vi "Process Incoming Messages by PDU F.vi"(0 "J1939 Cluster":T11, 1 "Conv Ref":T2, 2 "Data Ref":T1, 5 "CAN frame":T9 {"payload" format="%x"; "timestamp" format="%<%.7X\n%x>T"; "type" items=["CAN Data"=0, "CAN Remote"=1, "CAN Bus Error"=2, "Delay"=224, "Log Trigger"=225, "Start Trigger"=226]; "identifier" format="%x"}, 7 "ref in":T3, 9 "Addresses":u8[](array[numeric]), 11 "error in":errorcluster, 12 "Simulated Addresses LUT":variant) -> (15 "error out":errorcluster)   [LabVIEW 2013, in "J1939 Addon Engine.lvlib"]
uses:
  Engine/J1939 Addon Engine.lvlib
  Types/Setup Information Cluster.ctl
  <vilib>/xnet/xnet.llb/XNET Frame CAN.ctl
  <vilib>/xnet/xnet.llb/XNET Frame Type CAN.ctl
  J1939 Utilities/Types/CAN Outgoing Message Cluster.ctl
  Types/TP List References.ctl
  Types/BAM Buffer Connections List_Ref.ctl
  Types/Connection Mode Generation Connection Ref.ctl
  Types/BAM Generation Connections List_Ref.ctl
  Types/Address Table Reference.ctl
  Types/RQST Lookup Table Reference.ctl
  Engine/Types/Conversion Lookup Table Reference.ctl
  Engine/Types/Data Lookup Table Reference.ctl
  J1939 Utilities/Types/PGN Fields Cluster.ctl
  Engine/Types/Simulated Settings.ctl
  Types/Compiled Simulated Settings.ctl
  Types/Monitor Settings.ctl
  <vilib>/NI Veristand/Custom Device API/Block Data Reference.ctl
  <vilib>/NI Veristand/Custom Device API/Data Reference.ctl
  Engine/Types/DTC FIFOs.ctl
  Types/TP Connections List State.ctl
  Types/Connection Mode Buffer Create New TP Connection State.ctl
  Types/Address Lookup Table Action.ctl
  Types/Address Lookup Table Data.ctl
  J1939 Utilities/SubVIs/Convert CAN Arb ID to J1939 ID.vi
  J1939 Utilities/SubVIs/Convert J1939 ID to CAN Arb ID.vi
  J1939 Utilities/SubVIs/Acknowledgement.vi
  Buffer Connections List_Actions.vi
  TP Buffer Search for Connection (No PGN).vi
  TP Buffer Add New Data Packet to Connection.vi
  TP Buffer Convert Connection Info to CAN Frame.vi
  TP Buffer Create New TP Connection.vi
  Connection Mode Generation Connections List_Actions.vi
  Connection Mode Generation Search for Connection (Remote Message).vi
  TP Buffer Search for Connection.vi
  Engine/SubVIs/Convert Data to DTC Frame.vi
  Engine/SubVIs/Conversion Lookup Table Get Conversion Parameter.vi
  Engine/SubVIs/Data Lookup Table Get Signals (Range).vi
  J1939 Utilities/SubVIs/Convert PGN + SA to J1939 ID.vi
  <vilib>/xnet/xnet.llb/XNET Convert.vi
  <vilib>/xnet/xnet.llb/XNET Convert (Signal to Frame Raw).vi
  J1939 Utilities/SubVIs/TP.CM EndofMsgACK.vi
  J1939 Utilities/SubVIs/TP.CM CTS.vi
  J1939 Utilities/SubVIs/TP.Conn Abort.vi
  Connection Mode Generation CTS Received.vi
  J1939 Utilities/SubVIs/Convert CAN Data (U32) to U8.vi
  J1939 Utilities/J1939 Utilities.lvlib
  J1939 Addon Shared.lvlib
  <vilib>/NI Veristand/Custom Device API/Custom Device API.lvlib
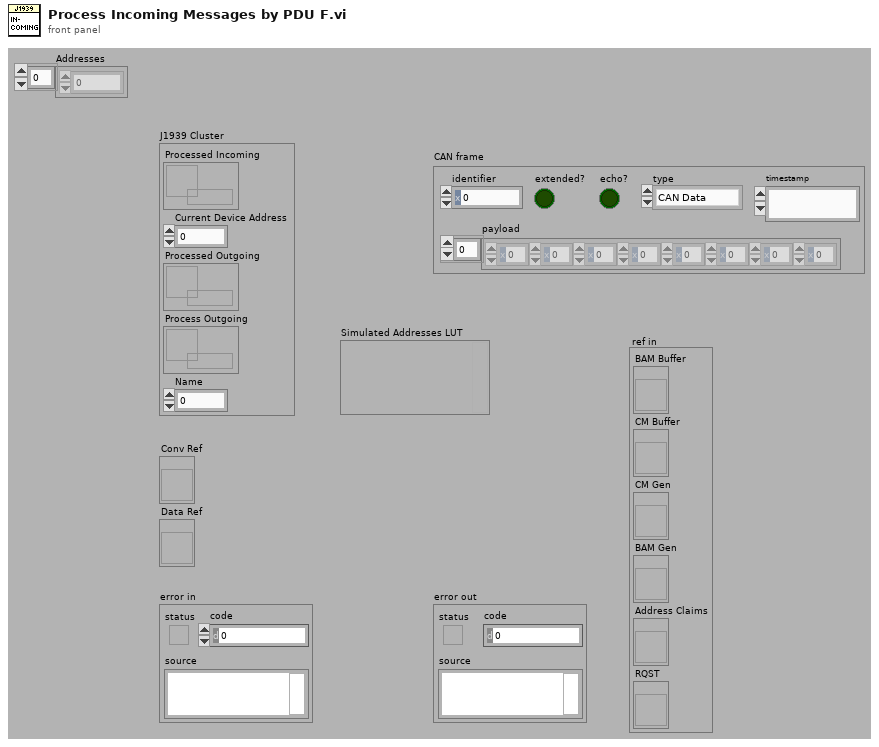
[diagram p1: front panel]
types:
  T1 = typedef "J1939 Addon Engine.lvlib/Data Lookup Table Reference.ctl" = refnum<vi>
  T2 = typedef "J1939 Addon Engine.lvlib/Conversion Lookup Table Reference.ctl" = refnum<vi>
  T3 = typedef "J1939 Addon Engine.lvlib/TP List References.ctl" = cluster{"BAM Buffer":T4, "CM Buffer":T4, "CM Gen":T5, "BAM Gen":T6, "Address Claims":T7, "RQST":T8}
  T4 = typedef "J1939 Addon Engine.lvlib/BAM Buffer Connections List_Ref.ctl" = refnum<vi>
  T5 = typedef "J1939 Addon Engine.lvlib/Connection Mode Generation Connection Ref.ctl" = refnum<vi>
  T6 = typedef "J1939 Addon Engine.lvlib/BAM Generation Connections List_Ref.ctl" = refnum<vi>
  T7 = typedef "J1939 Addon Engine.lvlib/Address Table Reference.ctl" = refnum<vi>
  T8 = typedef "J1939 Addon Engine.lvlib/RQST Lookup Table Reference.ctl" = refnum<vi>
  T9 = typedef "XNET Frame CAN.ctl" = cluster{"timestamp":timestamp, "payload":u8[], "identifier":u32, "type":T10, "extended?":bool, "echo?":bool}
  T10 = typedef "XNET Frame Type CAN.ctl" = u8
  T11 = typedef "J1939 Addon Engine.lvlib/Setup Information Cluster.ctl" = cluster{"Processed Incoming":refnum<queue>, "Current Device Address":u8, "Processed Outgoing":refnum<queue>, "Process Outgoing":refnum<queue>, "Name":u64}
  T12 = typedef "J1939 Addon Shared.lvlib/J1939 Utilities.lvlib/Message Types.ctl" = enum8{"PDU 1", "RQST2", "XFER", "ACKM", "RQST", "TP.DT - RTS/CTS", "TP.DT - BAM", "TP.CM - RTS", "TP.CM - CTS", "TP.CM - EndofMsgACK", "TP.CM - BAM", "TP.CM - Abort", "TP.CM - Error", "ACL", "Proprietary A", "PDU 2", "Proprietary B", "Error"}
  T13 = typedef "J1939 Addon Engine.lvlib/Simulated Settings.ctl" = cluster{"Simulated Addresses":T14, "FIFOs":T18}
  T14 = typedef "J1939 Addon Shared.lvlib/Compiled Simulated Settings.ctl" = cluster{"J1939 XNET Settings":T15, "DM1 Data":T16[], "DM1 Data":dbl[], "DM1 Active?":T16[], "DM1 Active?":dbl[], "DM2 Data":T16[], "DM2 Data":dbl[], "DM2 Active?":T16[], "DM2 Active?":dbl[]}
  T15 = typedef "J1939 Addon Shared.lvlib/Monitor Settings.ctl" = cluster{"J1939 Network Address":u8, "Name":u64}
  T16 = typedef "Custom Device API.lvlib/Block Data Reference.ctl" = cluster{"Data Reference":T17, "Offset":i32, "Length":i32}
  T17 = typedef "Custom Device API.lvlib/Data Reference.ctl" = i32
  T18 = typedef "J1939 Addon Engine.lvlib/DTC FIFOs.ctl" = cluster{"DM1 Data":refnum<k33>, "DM1 Active?":refnum<k33>, "DM2 Data":refnum<k33>, "DM2 Active?":refnum<k33>, "DM1 Reset?":refnum<k33>, "DM2 Reset?":refnum<k33>}
  T19 = typedef "J1939 Addon Shared.lvlib/J1939 Utilities.lvlib/PGN Fields Cluster.ctl" = cluster{"Reserved Bit":u8, "Data page":u8, "PDU Format":u8, "PDU Specific":u8}
  T20 = typedef "J1939 Addon Shared.lvlib/J1939 Utilities.lvlib/CAN Outgoing Message Cluster.ctl" = cluster{"Identifier":u32, "Data":u8[]}
  T21 = typedef "J1939 Addon Engine.lvlib/TP Connections List State.ctl" = enum16{"Add", "Update", "Get", "Remove", "Initialize"}
  T22 = typedef "J1939 Addon Engine.lvlib/Connection Mode Buffer Create New TP Connection State.ctl" = enum8{"Find Connection", "Create Connection", "Create CTS Frame", "Abort New Connection"}
  T23 = typedef "J1939 Addon Shared.lvlib/Address Lookup Table Data.ctl" = cluster{"Name":u8[], "Address":u8}
  T24 = typedef "J1939 Addon Engine.lvlib/Address Lookup Table Action.ctl" = enum16{"Initialize", "Add", "Get", "Remove", "Get All"}
  T25 = typedef "J1939 Addon Engine.lvlib/RQST Lookup Table Cluster.ctl" = cluster{"Response Q":refnum<queue>, "Request PGN":u32}
  T26 = typedef "J1939 Addon Shared.lvlib/J1939 Utilities.lvlib/Convert CAN Data (U8) Cluster.ctl" = cluster{"Byte 1":u8, "Byte 2":u8, "Byte 3":u8, "Byte 4":u8, "Byte 5":u8, "Byte 6":u8, "Byte 7":u8, "Byte 8":u8}
  T27 = typedef "J1939 Addon Engine.lvlib/TP Buffer Connection Cluster.ctl" = cluster{"Source Address":u8, "Destination Address":u8, "PGN":u32, "Arb ID":u32, "CAN Conversion Index":u32, "Total Expected Bytes":u16, "Total Expected Packets":u8, "Number of Packets Read":u8, "Start Time":u32, "Packets (U8)":u8[], "Timestamp":timestamp}
  T28 = typedef "J1939 Addon Engine.lvlib/Connection Mode Generation Connection Cluster.ctl" = cluster{"Total Packets":u8, "Current Packet to Generate":u8, "Packets":T20[], "Previous Time Stamp":u32, "Total Bytes":u16, "Packet Identifier [PDU S + SA]":u16, "Number of Packets to Generate":u8, "PGN":u32}
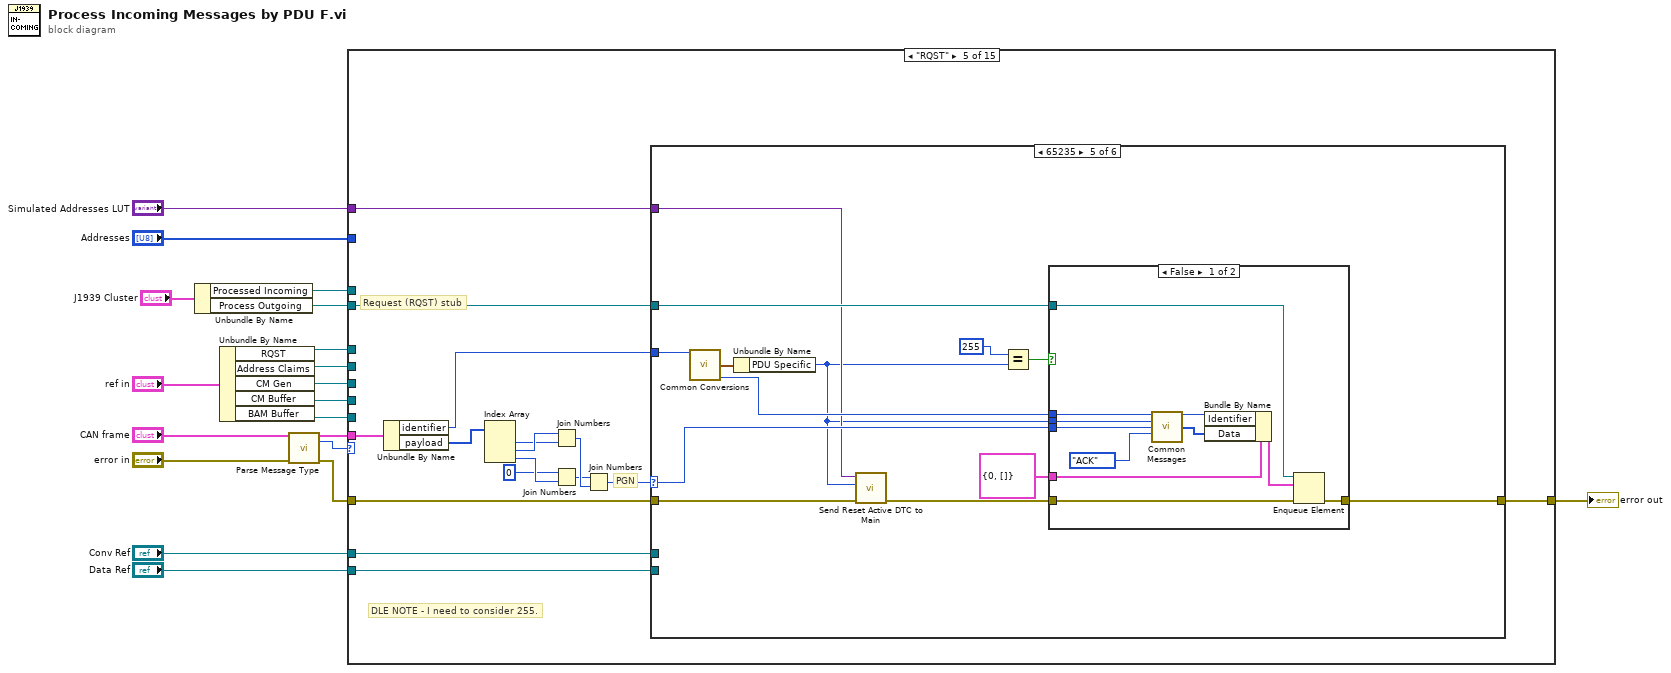
[diagram p0: block diagram]
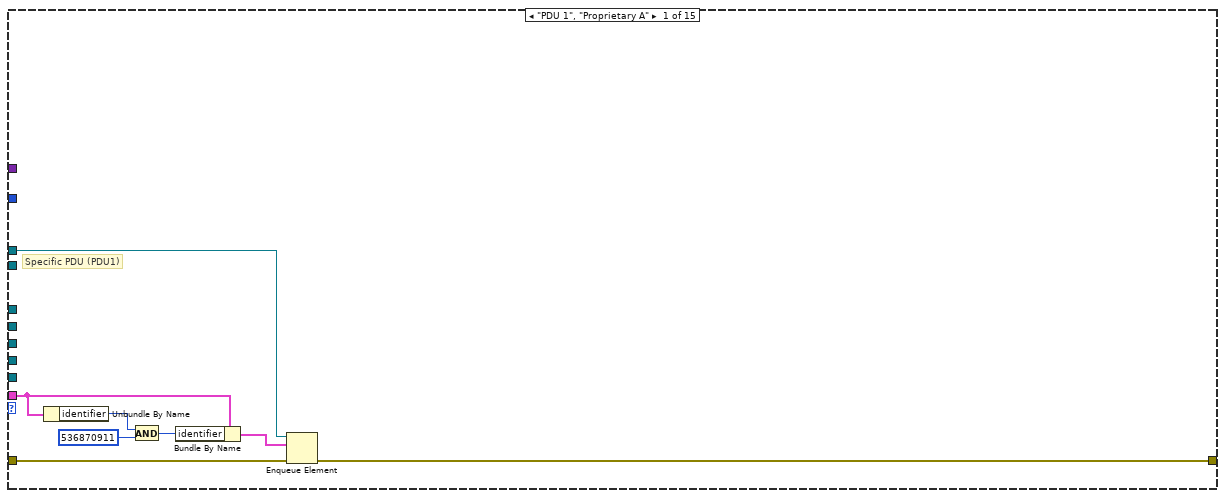
[diagram p2: hidden frame]
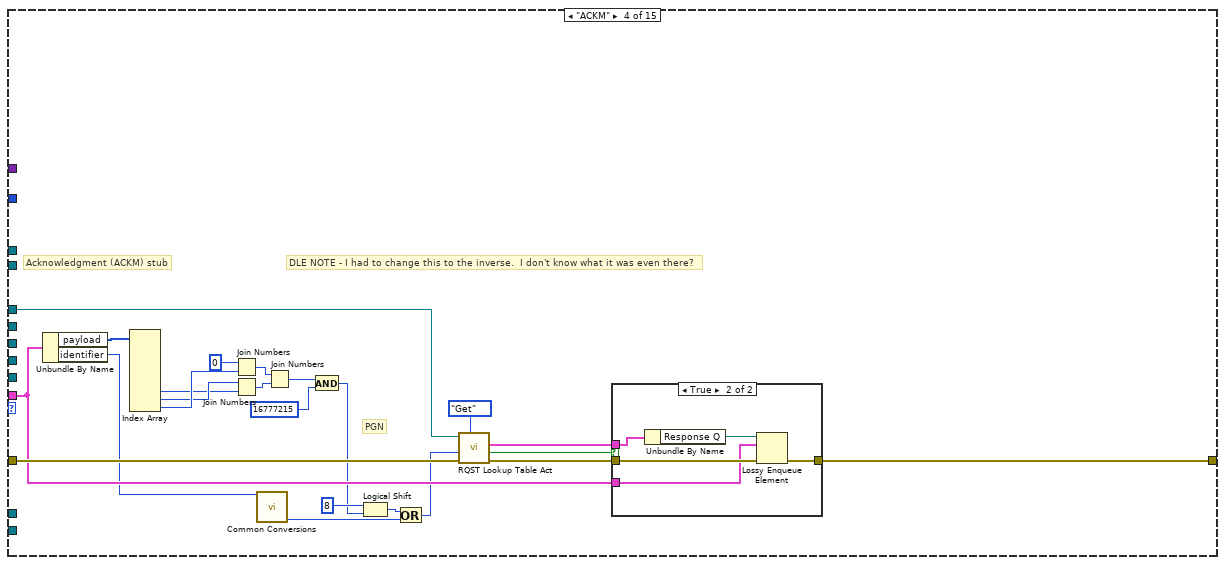
[diagram p5: hidden frame]
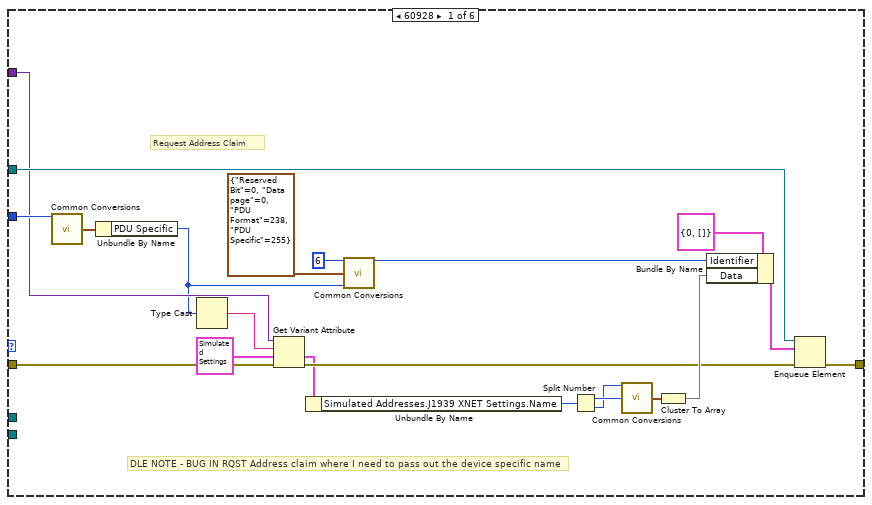
[diagram p7: hidden frame]
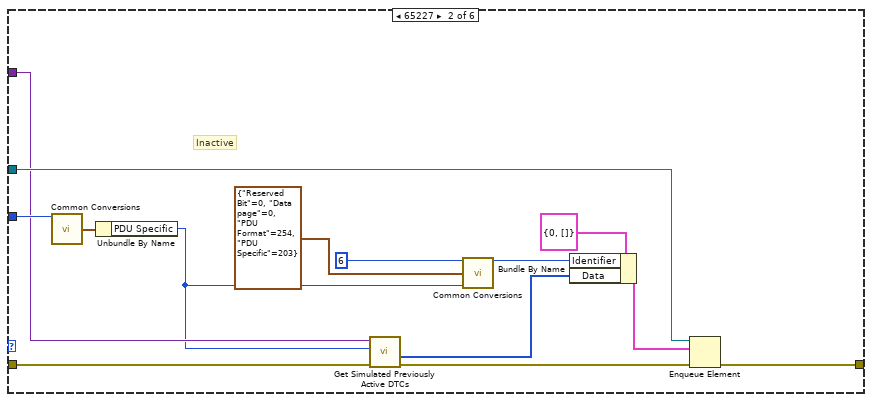
[diagram p8: hidden frame]
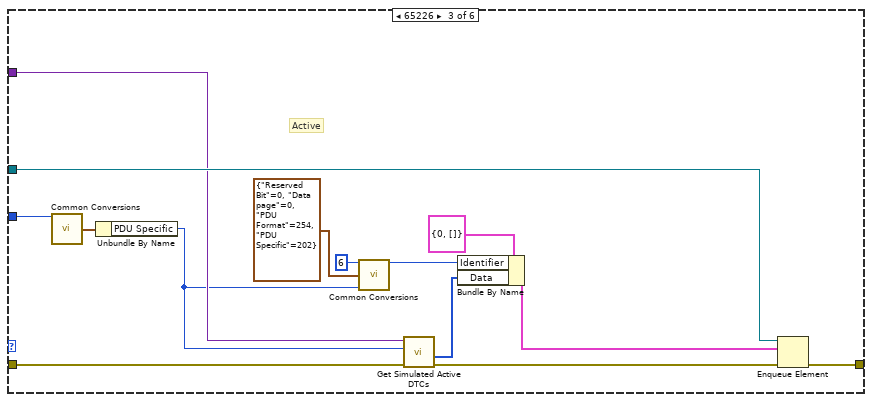
[diagram p9: hidden frame]
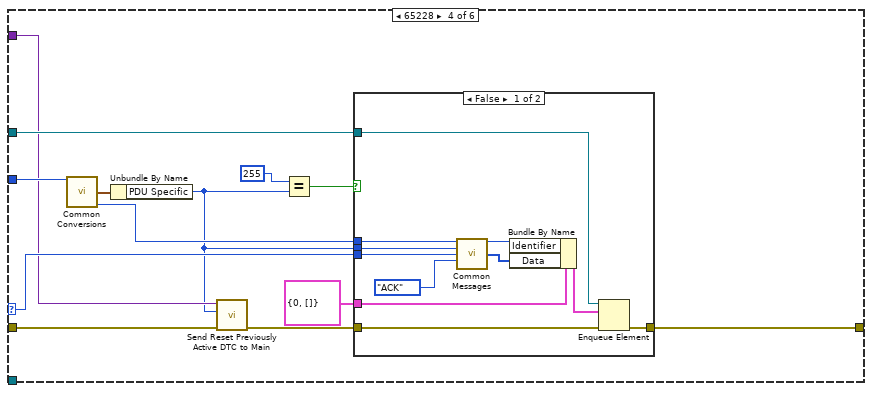
[diagram p10: hidden frame]
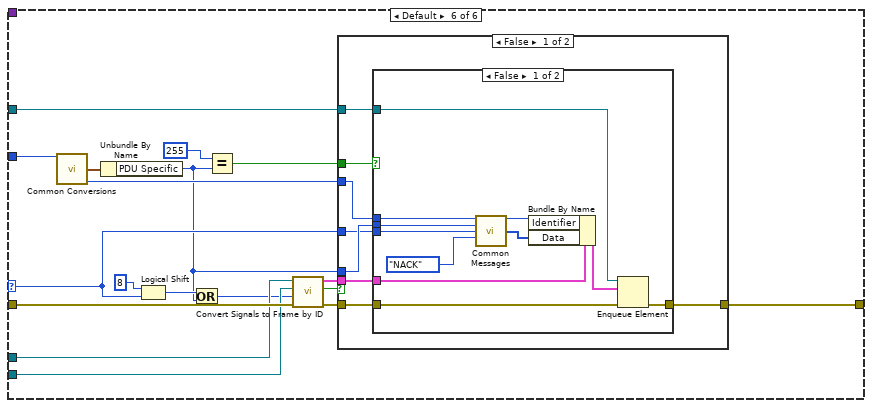
[diagram p13: hidden frame]
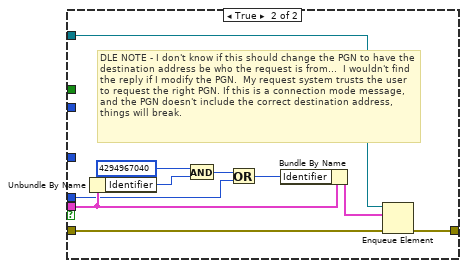
[diagram p15: hidden frame]
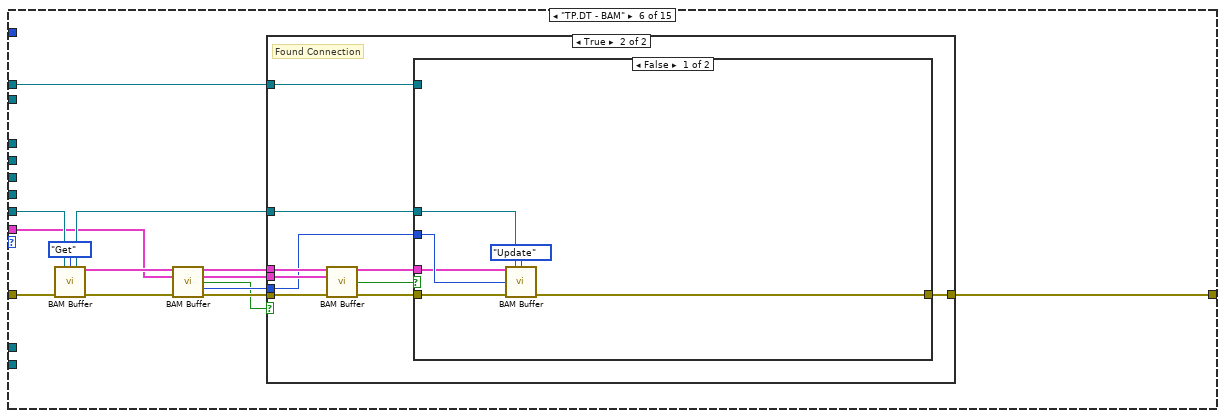
[diagram p16: hidden frame]
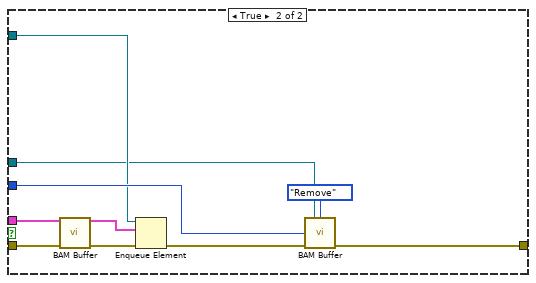
[diagram p18: hidden frame]
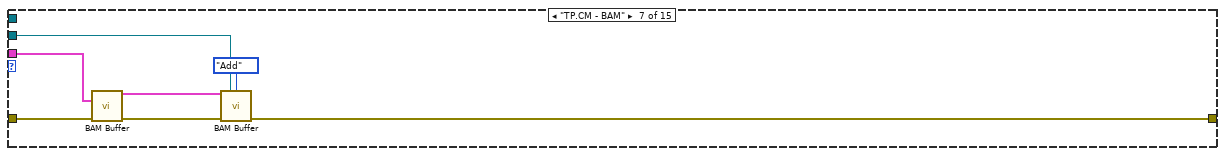
[diagram p19: hidden frame]
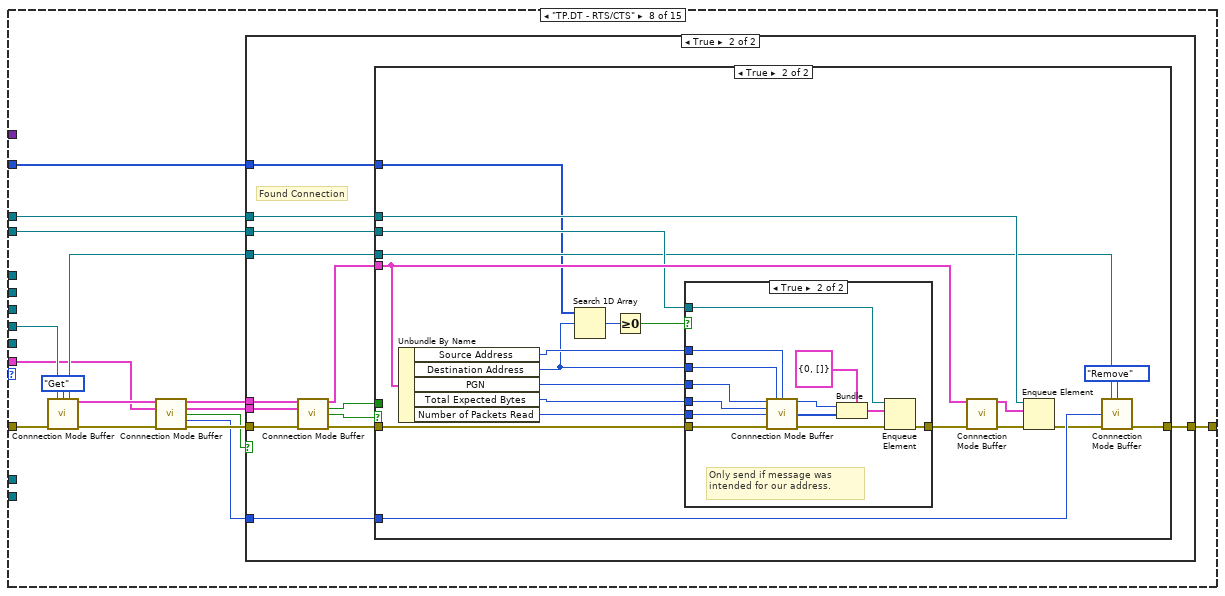
[diagram p20: hidden frame]
diagram:
  n1 = Unbundle By Name("J1939 Cluster") -> ("Processed Incoming"=w13:refnum<queue>, "Process Outgoing"=w12:refnum<queue>)
  n2 = Unbundle By Name("ref in") -> ("RQST"=w6:T8, "Address Claims"=w7:T7, "CM Gen"=w8:T5, "CM Buffer"=w9:T4, "BAM Buffer"=w10:T4)
  n3 = call "Parse Message Type.vi"("CAN frame"="CAN frame", "error in"="error in") -> ("CAN frame"=w16:T9, "State"=w15:T12, "error out"=w17:errorcluster)  [unwired: 1 in, 10 out]
  n4 = case shown="\"RQST\"" w15 {
    tunnel: w17 -> [w27 w28 w29 w39 w65 w228 w269 w285 w352 w454 w495 w511 w547 w559 w565]
    tunnel: [w26 w28 w29 w40 w66 w230 w266 w278 w351 w453 w494 w512 w540 w560 w565] -> w19
    tunnel: w16 -> [w22 _ _ w38 w74 w222 w263 w272 w348 w442 w485 w502 w538 w557 _]
    tunnel: w13 -> [w25 _ _ _ _ w225 _ w276 _ _ _ _ w537 w558 _]
    tunnel: w12 -> [_ _ _ _ w64 _ _ w275 w350 _ _ _ _ _ _]
    tunnel: w10 -> [_ _ _ _ _ w224 w264 _ _ _ _ _ _ _ _]
    tunnel: w9 -> [_ _ _ _ _ _ _ w274 w349 w441 _ w505 _ _ _]
    tunnel: w8 -> [_ _ _ _ _ _ _ _ _ w444 w487 w503 _ _ _]
    tunnel: w7 -> [_ _ _ _ _ _ _ _ _ _ _ _ w545 _ _]
    tunnel: w6 -> [_ _ _ w30 _ _ _ _ _ _ _ _ _ _ _]
    tunnel: "Conv Ref" -> [_ _ _ _ w62 _ _ _ _ _ _ _ _ _ _]
    tunnel: "Data Ref" -> [_ _ _ _ w61 _ _ _ _ _ _ _ _ _ _]
    tunnel: "Addresses" -> [_ _ _ _ _ _ _ w270 w347 _ _ _ _ _ _]
    tunnel: "Simulated Addresses LUT" -> [_ _ _ _ w59 _ _ _ _ _ _ _ _ _ _]
    frame "PDU 1", "Proprietary A" {
      # "Specific PDU (PDU1)"
      n5 = Unbundle By Name(w22) -> ("identifier"=w24:u32)
      n6 = And(x=w24, y=u32 536870911) -> (x .and. y?=w20:u32)
      n7 = Bundle By Name(cluster=w22, "identifier"=w20) -> (w21:T9)
      n8 = Enqueue Element(queue=w25, element=w21, error in (no error)=w27) -> (error out=w26:errorcluster)  [unwired: 3 out]
    }
    frame "RQST2" {
      # "Request2 (RQST2) Stub"
    }
    frame "XFER" {
      # "Transfer (XFER) Stub"
    }
    frame "ACKM" {
      # "DLE NOTE - I had to change this to the inverse.  I don't know what it was even there?"
      # "PGN"
      # "Acknowledgment (ACKM) stub"
      n9 = Unbundle By Name(w38) -> ("payload"=w52:u8[], "identifier"=w35:u32)
      n10 = Index Array(array=w52) -> (element #6=w49:u8, element #7=w50:u8, element #8=w51:u8)  [unwired: 8 in, 5 out]
      n11 = Join Numbers(hi=u8 0, lo=w51) -> ((hi.lo)=w48:u16)
      n12 = Join Numbers(hi=w50, lo=w49) -> ((hi.lo)=w47:u16)
      n13 = call-poly "Common Conversions.vi"("Arb ID"=w35) -> ("Source Address"=w34:u8)  [unwired: 11 in, 3 out]
      n14 = Join Numbers(hi=w48, lo=w47) -> ((hi.lo)=w46:u32)
      n15 = And(x=w46, y=u32 16777215 ("x")) -> (x .and. y?=w33:u32)
      n16 = Logical Shift(y=i8 8, x=w33) -> (x << y=w37:u32)
      n17 = Or(x=w37, y=w34) -> (x .or. y?=w32:u32)
      n18 = call "RQST Lookup Table Act.vi"("Action"=enum16{"Initialize", "Add", "Get", "Remove"}."Get", "error in (no error)"=w39, "ID"=w32, "ref in"=w30) -> ("error out"=w31:errorcluster, "Found?"=w42:bool, "Data"=w41:T25)  [unwired: 5 in]
      n19 = case shown="True" w42 {
        tunnel: w41 -> [_ w57]
        tunnel: w31 -> [w53 w58]
        tunnel: w38 -> [_ w55]
        tunnel: [w53 w54] -> w40
        frame False {
        }
        frame True {
          n20 = Unbundle By Name(w57) -> ("Response Q"=w56:refnum<queue>)
          n21 = Lossy Enqueue Element(queue=w56, element=w55, error in (no error)=w58) -> (error out=w54:errorcluster)  [unwired: 3 out]
        }
      }
    }
    frame "RQST" {
      # "DLE NOTE - I need to consider 255."
      # "PGN"
      # "Request (RQST) stub"
      n22 = Unbundle By Name(w74) -> ("identifier"=w63:u32, "payload"=w73:u8[])
      n23 = Index Array(array=w73) -> (element #1=w60:u8, element #2=w72:u8, element #3=w71:u8)  [unwired: 3 in]
      n24 = Join Numbers(hi=w72, lo=w60) -> ((hi.lo)=w69:u16)
      n25 = Join Numbers(hi=u8 0, lo=w71) -> ((hi.lo)=w68:u16)
      n26 = Join Numbers(hi=w68, lo=w69) -> ((hi.lo)=w67:u32)
      n27 = case shown="65235" w67 {
        selector: w67 -> [_ _ _ w130 w155 w181]
        tunnel: [w91 w102 w117 w131 w153 w182] -> w66
        tunnel: w65 -> [w78 w98 w111 w127 w152 w191]
        tunnel: w64 -> [w89 w101 w116 w132 w156 w183]
        tunnel: w63 -> [w83 w108 w122 w135 w154 w184]
        tunnel: w62 -> [_ _ _ _ _ w190]
        tunnel: w61 -> [_ _ _ _ _ w189]
        tunnel: w59 -> [w80 w100 w113 w125 w150 _]
        frame 60928 {
          # "DLE NOTE - BUG IN RQST Address claim where I need to pass out the device specific name"
          # "Request Address Claim"
          n28 = call-poly "Common Conversions.vi"("Arb ID"=w83) -> ("PGN Fields"=w84:T19)  [unwired: 11 in, 3 out]
          n29 = Unbundle By Name(w84) -> ("PDU Specific"=w79:u8)
          n30 = Type Cast(x=w79) -> (*(type *) &x=w81:string)  [unwired: 1 in]
          n31 = Get Variant Attribute(Variant=w80, name=w81, default value (empty Variant)=T13 {"Simulated Addresses"={"J1939 XNET Settings"={"J1939 Network Address"=0, "Name"=0}, "DM1 Data"=[], "DM1 Data"=[], "DM1 Active?"=[], "DM1 Active?"=[], "DM2 Data"=[], "DM2 Data"=[], "DM2 Active?"=[], "DM2 Active?"=[]}, "FIFOs"={"DM1 Data"=refnum, "DM1 Active?"=refnum, "DM2 Data"=refnum, "DM2 Active?"=refnum, "DM1 Reset?"=refnum, "DM2 Reset?"=refnum}} ("Cluster"), error in=w78) -> (value=w76:T13, error out=w77:errorcluster)  [unwired: 2 out]
          n32 = Unbundle By Name(w76) -> ("Simulated Addresses.J1939 XNET Settings.Name"=w75:u64)
          n33 = call-poly "Common Conversions.vi"("Priority"=u8 6, "PGN Fields"=T19 {"Reserved Bit"=0, "Data page"=0, "PDU Format"=238, "PDU Specific"=255}, "Source Address"=w79) -> ("ID"=w93:u32)  [unwired: 2 in, 10 out]
          n34 = Split Number(x=w75) -> (hi(x)=w87:u32, lo(x)=w86:u32)
          n35 = call-poly "Common Conversions.vi"("Data 0-3"=w86, "Data 4-7"=w87) -> ("Byte Cluster"=w88:T26)  [unwired: 13 in]
          n36 = Cluster To Array(cluster=w88) -> (array=w85:u8[])
          n37 = Bundle By Name(cluster=T20 {"Identifier"=0, "Data"=[]} ("Data to Send"), "Identifier"=w93, "Data"=w85) -> (w90:T20)
          n38 = Enqueue Element(queue=w89, element=w90, error in (no error)=w77) -> (error out=w91:errorcluster)  [unwired: 1 in, 2 out]
        }
        frame 65227 {
          # "Inactive"
          n39 = call-poly "Common Conversions.vi"("Arb ID"=w108) -> ("PGN Fields"=w109:T19)  [unwired: 11 in, 3 out]
          n40 = Unbundle By Name(w109) -> ("PDU Specific"=w99:u8)
          n41 = call "Get Simulated Previously Active DTCs.vi"("error in (no error)"=w98, "Address"=w99, "Simulated Addresses LUT"=w100) -> ("error out"=w97:errorcluster, "DTC Frame"=w96:u8[])  [unwired: 6 in, 1 out]
          n42 = call-poly "Common Conversions.vi"("Priority"=u8 6, "PGN Fields"=T19 {"Reserved Bit"=0, "Data page"=0, "PDU Format"=254, "PDU Specific"=203}, "Source Address"=w99) -> ("ID"=w105:u32)  [unwired: 2 in, 10 out]
          n43 = Bundle By Name(cluster=T20 {"Identifier"=0, "Data"=[]} ("Data to Send"), "Identifier"=w105, "Data"=w96) -> (w107:T20)
          n44 = Enqueue Element(queue=w101, element=w107, error in (no error)=w97) -> (error out=w102:errorcluster)  [unwired: 1 in, 2 out]
        }
        frame 65226 {
          # "Active"
          n45 = call-poly "Common Conversions.vi"("Arb ID"=w122) -> ("PGN Fields"=w123:T19)  [unwired: 11 in, 3 out]
          n46 = Unbundle By Name(w123) -> ("PDU Specific"=w112:u8)
          n47 = call-poly "Common Conversions.vi"("Priority"=u8 6, "PGN Fields"=T19 {"Reserved Bit"=0, "Data page"=0, "PDU Format"=254, "PDU Specific"=202}, "Source Address"=w112) -> ("ID"=w119:u32)  [unwired: 2 in, 10 out]
          n48 = call "Get Simulated Active DTCs.vi"("error in (no error)"=w111, "Address"=w112, "Simulated Addresses LUT"=w113) -> ("error out"=w114:errorcluster, "DTC Frame"=w110:u8[])  [unwired: 6 in, 1 out]
          n49 = Bundle By Name(cluster=T20 {"Identifier"=0, "Data"=[]} ("Data to Send"), "Identifier"=w119, "Data"=w110) -> (w121:T20)
          n50 = Enqueue Element(queue=w116, element=w121, error in (no error)=w114) -> (error out=w117:errorcluster)  [unwired: 1 in, 2 out]
        }
        frame 65228 {
          n51 = call-poly "Common Conversions.vi"("Arb ID"=w135) -> ("PGN Fields"=w136:T19, "Source Address"=w129:u8)  [unwired: 11 in, 2 out]
          n52 = Unbundle By Name(w136) -> ("PDU Specific"=w124:u8)
          n53 = call "Send Reset Previously Active DTC to Main.vi"("error in (no error)"=w127, "Address"=w124, "Simulated Addresses LUT"=w125) -> ("error out"=w126:errorcluster)  [unwired: 7 in, 1 out]
          n54 = Equal?(x=u8 255 ("y"), y=w124) -> (x = y?=w133:bool)
          n55 = case shown="False" w133 {
            tunnel: w126 -> [w147 w148]
            tunnel: [w146 w148] -> w131
            tunnel: w132 -> [w145 _]
            tunnel: w129 -> [w144 _]
            tunnel: w124 -> [w143 _]
            tunnel: w130 -> [w142 _]
            tunnel: T20 {"Identifier"=0, "Data"=[]} ("Frame") -> [w140 _]
            frame False {
              n56 = call-poly "Common Messages.vi"("Destination Address"=w144, "Source Address"=w143, "PGN"=w142, "Control Byte"=enum8{"ACK", "NACK", "Access Denied"}."ACK") -> ("Arb ID"=w139:u32, "Data"=w138:u8[])  [unwired: 10 in]
              n57 = Bundle By Name(cluster=w140, "Identifier"=w139, "Data"=w138) -> (w137:T20)
              n58 = Enqueue Element(queue=w145, element=w137, error in (no error)=w147) -> (error out=w146:errorcluster)  [unwired: 3 out]
            }
            frame True {
            }
          }
        }
        frame 65235 {
          n59 = call-poly "Common Conversions.vi"("Arb ID"=w154) -> ("PGN Fields"=w161:T19, "Source Address"=w158:u8)  [unwired: 11 in, 2 out]
          n60 = Unbundle By Name(w161) -> ("PDU Specific"=w149:u8)
          n61 = call "Send Reset Active DTC to Main.vi"("error in (no error)"=w152, "Address"=w149, "Simulated Addresses LUT"=w150) -> ("error out"=w151:errorcluster)  [unwired: 7 in, 1 out]
          n62 = Equal?(x=u8 255 ("y"), y=w149) -> (x = y?=w159:bool)
          n63 = case shown="False" w159 {
            tunnel: w151 -> [w172 w173]
            tunnel: [w171 w173] -> w153
            tunnel: w156 -> [w170 _]
            tunnel: w158 -> [w169 _]
            tunnel: w149 -> [w168 _]
            tunnel: w155 -> [w167 _]
            tunnel: T20 {"Identifier"=0, "Data"=[]} ("Frame") -> [w165 _]
            frame False {
              n64 = call-poly "Common Messages.vi"("Destination Address"=w169, "Source Address"=w168, "PGN"=w167, "Control Byte"=enum8{"ACK", "NACK", "Access Denied"}."ACK") -> ("Arb ID"=w164:u32, "Data"=w163:u8[])  [unwired: 10 in]
              n65 = Bundle By Name(cluster=w165, "Identifier"=w164, "Data"=w163) -> (w162:T20)
              n66 = Enqueue Element(queue=w170, element=w162, error in (no error)=w172) -> (error out=w171:errorcluster)  [unwired: 3 out]
            }
            frame True {
            }
          }
        }
        frame Default {
          n67 = call-poly "Common Conversions.vi"("Arb ID"=w184) -> ("PGN Fields"=w180:T19, "Source Address"=w177:u8)  [unwired: 11 in, 2 out]
          n68 = Unbundle By Name(w180) -> ("PDU Specific"=w174:u8)
          n69 = Logical Shift(y=i8 8, x=w181) -> (x << y=w176:u32)
          n70 = Or(x=w176, y=w174) -> (x .or. y?=w175:u32)
          n71 = Equal?(x=u8 255 ("y"), y=w174) -> (x = y?=w178:bool)
          n72 = call "Convert Signals to Frame by ID.vi"("error in (no error)"=w191, "ID"=w175, "Data Ref"=w189, "Conv Ref"=w190) -> ("error out"=w185:errorcluster, "Found?"=w186:bool, "Frame"=w187:T20)  [unwired: 5 in]
          n73 = case shown="False" w186 {
            tunnel: w187 -> [w193 w221]
            tunnel: w174 -> [w195 w219]
            tunnel: [w198 w214] -> w182
            tunnel: w185 -> [w199 w215]
            tunnel: w177 -> [w196 _]
            tunnel: w183 -> [w197 w216]
            tunnel: w181 -> [w194 _]
            tunnel: w178 -> [w192 _]
            frame False {
              n74 = case shown="False" w192 {
                tunnel: w199 -> [w210 w211]
                tunnel: [w209 w211] -> w198
                tunnel: w197 -> [w208 _]
                tunnel: w196 -> [w207 _]
                tunnel: w195 -> [w206 _]
                tunnel: w194 -> [w205 _]
                tunnel: w193 -> [w203 _]
                frame False {
                  n75 = call-poly "Common Messages.vi"("Destination Address"=w207, "Source Address"=w206, "PGN"=w205, "Control Byte"=enum8{"ACK", "NACK", "Access Denied"}."NACK") -> ("Arb ID"=w202:u32, "Data"=w201:u8[])  [unwired: 10 in]
                  n76 = Bundle By Name(cluster=w203, "Identifier"=w202, "Data"=w201) -> (w200:T20)
                  n77 = Enqueue Element(queue=w208, element=w200, error in (no error)=w210) -> (error out=w209:errorcluster)  [unwired: 3 out]
                }
                frame True {
                }
              }
            }
            frame True {
              # "DLE NOTE - I don't know if this should change the PGN to have the destination address be who the request is from...  I wouldn't find the reply if I modify the PGN.  My request system trusts the user to request the right PGN. If this is a connection mode message, and the PGN doesn't include the correct destination address, things will break."
              n78 = Unbundle By Name(w221) -> ("Identifier"=w220:u32)
              n79 = And(x=u32 4294967040 ("y"), y=w220) -> (x .and. y?=w212:u32)
              n80 = Or(x=w212, y=w219) -> (x .or. y?=w218:u32)
              n81 = Bundle By Name(cluster=w221, "Identifier"=w218) -> (w217:T20)
              n82 = Enqueue Element(queue=w216, element=w217, error in (no error)=w215) -> (error out=w214:errorcluster)  [unwired: 3 out]
            }
          }
        }
      }
    }
    frame "TP.DT - BAM" {
      n83 = call-poly "BAM Buffer.vi"("ref in"=w224, "State"=TP_Connections_List_State."Get", "error in (no error)"=w228) -> ("ref out"=w223:T4, "Connections"=w234:T27[], "error out"=w227:errorcluster)  [unwired: 2 in, 8 out]
      n84 = call-poly "BAM Buffer.vi"("Connecctions"=w234, "CAN frame"=w222, "error in (no error)"=w227) -> ("Connection Cluster Out"=w233:T27, "CAN frame Out"=w232:T9, "Found?"=w226:bool, "Index"=w229:i32, "error out"=w231:errorcluster)  [unwired: 8 out]
      n85 = case shown="True" w226 {
        tunnel: w233 -> [_ w246]
        tunnel: w232 -> [_ w244]
        tunnel: w231 -> [w236 w243]
        tunnel: [w236 w241] -> w230
        tunnel: w229 -> [_ w240]
        tunnel: w225 -> [_ w238]
        tunnel: w223 -> [_ w237]
        frame False {
        }
        frame True {
          # "Found Connection"
          n86 = call-poly "BAM Buffer.vi"("Connection Cluster"=w246, "CAN frame"=w244, "error in (no error)"=w243) -> ("Connection Cluster Out"=w239:T27, "Message Complete?"=w245:bool, "error out"=w242:errorcluster)  [unwired: 10 out]
          n87 = case shown="False" w245 {
            tunnel: w242 -> [w250 w260]
            tunnel: [w249 w258] -> w241
            tunnel: w240 -> [w251 w261]
            tunnel: w239 -> [w247 w259]
            tunnel: w238 -> [_ w255]
            tunnel: w237 -> [w248 w253]
            frame False {
              n88 = call-poly "BAM Buffer.vi"("Connection Cluster"=w247, "ref in"=w248, "State"=TP_Connections_List_State."Update", "index"=w251, "error in (no error)"=w250) -> ("error out"=w249:errorcluster)  [unwired: 7 in, 3 out]
            }
            frame True {
              n89 = call-poly "BAM Buffer.vi"("Connection Cluster"=w259, "error in (no error)"=w260) -> ("CAN frame"=w254:T9, "error out"=w257:errorcluster)  [unwired: 12 out]
              n90 = Enqueue Element(queue=w255, element=w254, error in (no error)=w257) -> (error out=w256:errorcluster)  [unwired: 3 out]
              n91 = call-poly "BAM Buffer.vi"("ref in"=w253, "State"=TP_Connections_List_State."Remove", "index"=w261, "error in (no error)"=w256) -> ("error out"=w258:errorcluster)  [unwired: 1 in, 10 out]
            }
          }
        }
      }
    }
    frame "TP.CM - BAM" {
      n92 = call-poly "BAM Buffer.vi"("CAN frame"=w263, "error in (no error)"=w269) -> ("Connection Cluster Out"=w265:T27, "error out"=w267:errorcluster)  [unwired: 1 in, 11 out]
      n93 = call-poly "BAM Buffer.vi"("Connection Cluster"=w265, "ref in"=w264, "State"=TP_Connections_List_State."Add", "error in (no error)"=w267) -> ("error out"=w266:errorcluster)  [unwired: 1 in, 10 out]
    }
    frame "TP.DT - RTS/CTS" {
      n94 = call-poly "Connnection Mode Buffer.vi"("ref in"=w274, "State"=TP_Connections_List_State."Get", "error in (no error)"=w285) -> ("ref out"=w273:T4, "Connections"=w283:T27[], "error out"=w282:errorcluster)  [unwired: 2 in, 8 out]
      n95 = call-poly "Connnection Mode Buffer.vi"("Connecctions"=w283, "CAN frame"=w272, "error in (no error)"=w282) -> ("Connection Cluster Out"=w280:T27, "CAN frame Out"=w277:T9, "Found?"=w271:bool, "Index"=w279:i32, "error out"=w281:errorcluster)  [unwired: 8 out]
      n96 = case shown="True" w271 {
        tunnel: w281 -> [w286 w299]
        tunnel: w280 -> [_ w298]
        tunnel: w277 -> [_ w297]
        tunnel: w279 -> [_ w294]
        tunnel: [w286 w293] -> w278
        tunnel: w276 -> [_ w292]
        tunnel: w275 -> [_ w289]
        tunnel: w273 -> [_ w288]
        tunnel: w270 -> [_ w287]
        frame False {
        }
        frame True {
          # "Found Connection"
          n97 = call-poly "Connnection Mode Buffer.vi"("Connection Cluster"=w298, "CAN frame"=w297, "error in (no error)"=w299) -> ("Connection Cluster Out"=w295:T27, "Frame Mismatch?"=w290:bool, "Message Complete?"=w291:bool, "error out"=w296:errorcluster)  [unwired: 9 out]
          n98 = case shown="True" w291 {
            tunnel: w296 -> [w305 w325]
            tunnel: [w304 w332] -> w293
            tunnel: w294 -> [w303 w331]
            tunnel: w295 -> [w302 w324]
            tunnel: w292 -> [_ w327]
            tunnel: w290 -> [w301 _]
            tunnel: w289 -> [_ w318]
            tunnel: w288 -> [w300 w317]
            tunnel: w287 -> [_ w315]
            frame False {
              n99 = case shown="False" w301 {
                tunnel: w305 -> [w310 w312]
                tunnel: [w309 w312] -> w304
                tunnel: w303 -> [w308 _]
                tunnel: w302 -> [w307 _]
                tunnel: w300 -> [w306 _]
                frame False {
                  n100 = call-poly "Connnection Mode Buffer.vi"("Connection Cluster"=w307, "ref in"=w306, "State"=TP_Connections_List_State."Update", "index"=w308, "error in (no error)"=w310) -> ("error out"=w309:errorcluster)  [unwired: 10 out]
                }
                frame True {
                }
              }
            }
            frame True {
              n101 = Unbundle By Name(w324) -> ("Source Address"=w323:u8, "Destination Address"=w314:u8, "PGN"=w322:u32, "Total Expected Bytes"=w320:u16, "Number of Packets Read"=w321:u8)
              n102 = Search 1D Array(1D array=w315, element=w314) -> (index of element=w313:i32)  [unwired: 1 in]
              n103 = Greater Or Equal To 0?(x=w313) -> (x >= 0?=w316:bool)
              n104 = case shown="True" w316 {
                tunnel: w325 -> [w333 w346]
                tunnel: w323 -> [_ w345]
                tunnel: w322 -> [_ w344]
                tunnel: w321 -> [_ w343]
                tunnel: w320 -> [_ w342]
                tunnel: [w333 w338] -> w319
                tunnel: w318 -> [_ w337]
                tunnel: w314 -> [_ w334]
                frame False {
                }
                frame True {
                  # "Only send if message was intended for our address."
                  n105 = call-poly "Connnection Mode Buffer.vi"("PGN"=w344, "Source Address"=w334, "Destination Address"=w345, "Total Message Size(bytes)"=w342, "Total Number of Packets"=w343, "error in (no error)"=w346) -> ("Arb ID"=w341:u32, "Data"=w340:u8[], "error out"=w339:errorcluster)  [unwired: 7 out]
                  n106 = Bundle(cluster=T20 {"Identifier"=0, "Data"=[]} ("Data to Send"), "Identifier"=w341, "Data"=w340) -> (w335:T20)
                  n107 = Enqueue Element(queue=w337, element=w335, error in (no error)=w339) -> (error out=w338:errorcluster)  [unwired: 3 out]
                }
              }
              n108 = call-poly "Connnection Mode Buffer.vi"("Connection Cluster"=w324, "error in (no error)"=w319) -> ("CAN frame"=w326:T9, "error out"=w329:errorcluster)  [unwired: 12 out]
              n109 = Enqueue Element(queue=w327, element=w326, error in (no error)=w329) -> (error out=w328:errorcluster)  [unwired: 3 out]
              n110 = call-poly "Connnection Mode Buffer.vi"("ref in"=w317, "State"=TP_Connections_List_State."Remove", "index"=w331, "error in (no error)"=w328) -> ("error out"=w332:errorcluster)  [unwired: 1 in, 10 out]
            }
          }
        }
      }
    }
    frame "TP.CM - RTS" {
      n111 = while {
        shift-right: [w358] -> _
        shift-left: Connection_Mode_Buffer_Create_New_TP_Connection_State."Find Connection" ("Action") -> [w365]
        tunnel: w348 -> [w366]
        shift-right: [w363] -> _
        shift-left: _ -> [w357]
        shift-right: [w362] -> _
        shift-left: _ -> [w359]
        shift-right: [w361] -> w351
        shift-left: w352 -> [w364]
        tunnel: w350 -> [w356]
        tunnel: w349 -> [w355]
        tunnel: w347 -> [w354]
        stop <- w360 stop-if-true
        n112 = case shown="\"Create CTS Frame\"" w365 {
          selector: w365 -> [_ _ w404 w423]
          tunnel: w366 -> [w377 w390 _ w422]
          tunnel: w364 -> [w376 w392 w407 w421]
          tunnel: [w375 w386 w406 w428] -> w363
          tunnel: [w374 w395 w405 w426] -> w362
          tunnel: [w373 w393 w401 w425] -> w361
          tunnel: [FALSE w385 TRUE TRUE] -> w360
          tunnel: w359 -> [_ w395 w405 w426]
          tunnel: [w369 Connection_Mode_Buffer_Create_New_TP_Connection_State."Create CTS Frame" ("Action") w404 w423] -> w358
          tunnel: w357 -> [_ _ w406 w428]
          tunnel: w356 -> [_ _ w400 w424]
          tunnel: w355 -> [w367 w387 _ _]
          tunnel: w354 -> [_ w383 _ w415]
          frame "Find Connection" {
            n113 = call-poly "Connnection Mode Buffer.vi"("ref in"=w367, "State"=TP_Connections_List_State."Get", "error in (no error)"=w376) -> ("Connections"=w379:T27[], "error out"=w380:errorcluster)  [unwired: 2 in, 9 out]
            n114 = call-poly "Connnection Mode Buffer.vi"("Connecctions"=w379, "CAN frame"=w377, "error in (no error)"=w380) -> ("Connection Cluster Out"=w375:T27, "Found?"=w370:bool, "Index"=w374:i32, "error out"=w373:errorcluster)  [unwired: 9 out]
            n115 = Select(t=Connection_Mode_Buffer_Create_New_TP_Connection_State."Abort New Connection", s=w370, f=Connection_Mode_Buffer_Create_New_TP_Connection_State."Create Connection" ("Action")) -> (s? t:f=w369:T22)
          }
          frame "Create Connection" {
            # "Stop if the intended address wasn't us."
            n116 = call-poly "Connnection Mode Buffer.vi"("CAN frame"=w390, "error in (no error)"=w392) -> ("Connection Cluster Out"=w389:T27, "error out"=w391:errorcluster)  [unwired: 12 out]
            n117 = call-poly "Connnection Mode Buffer.vi"("Connection Cluster"=w389, "ref in"=w387, "State"=TP_Connections_List_State."Add", "error in (no error)"=w391) -> ("Connection Cluster Out"=w386:T27, "error out"=w393:errorcluster)  [unwired: 1 in, 9 out]
            n118 = Unbundle By Name(w386) -> ("Destination Address"=w382:u8)
            n119 = Search 1D Array(1D array=w383, element=w382) -> (index of element=w384:i32)  [unwired: 1 in]
            n120 = Greater Or Equal To 0?(x=w384) -> (x >= 0?=w381:bool)
            n121 = Not(x=w381) -> (.not. x?=w385:bool)
          }
          frame "Create CTS Frame" {
            # "Only send if the message was intended for our address."
            n122 = Unbundle By Name(w406) -> ("Source Address"=w412:u8, "Destination Address"=w411:u8, "PGN"=w410:u32, "Total Expected Packets"=w408:u8)
            n123 = call-poly "Connnection Mode Buffer.vi"("PGN"=w410, "Source Address"=w411, "Destination Address"=w412, "Number of Packets to Send"=w408, "Next Packet to Send"=u8 1, "error in (no error)"=w407) -> ("Arb ID"=w399:u32, "Data"=w398:u8[], "error out"=w402:errorcluster)  [unwired: 1 in, 6 out]
            n124 = Bundle(cluster=T20 {"Identifier"=0, "Data"=[]} ("Data to Send"), "Identifier"=w399, "Data"=w398) -> (w396:T20)
            n125 = Enqueue Element(queue=w400, element=w396, error in (no error)=w402) -> (error out=w401:errorcluster)  [unwired: 3 out]
          }
          frame "Abort New Connection" {
            n126 = call-poly "Connnection Mode Buffer.vi"("CAN frame"=w422, "error in (no error)"=w421) -> ("Connection Cluster Out"=w419:T27, "error out"=w420:errorcluster)  [unwired: 12 out]
            n127 = Unbundle By Name(w419) -> ("Source Address"=w418:u8, "Destination Address"=w414:u8, "PGN"=w417:u32)
            n128 = Search 1D Array(1D array=w415, element=w414) -> (index of element=w416:i32)  [unwired: 1 in]
            n129 = Greater Or Equal To 0?(x=w416) -> (x >= 0?=w413:bool)
            n130 = case shown="False" w413 {
              tunnel: w420 -> [w429 w440]
              tunnel: [w429 w436] -> w425
              tunnel: w424 -> [_ w433]
              tunnel: w418 -> [_ w432]
              tunnel: w414 -> [_ w431]
              tunnel: w417 -> [_ w430]
              frame False {
              }
              frame True {
                n131 = call-poly "Connnection Mode Buffer.vi"("Destination Address"=w432, "Source Address"=w431, "PGN"=w430, "error in (no error)"=w440) -> ("Arb ID"=w439:u32, "Data"=w438:u8[], "error out"=w437:errorcluster)  [unwired: 2 in, 7 out]
                n132 = Bundle(cluster=T20 {"Identifier"=0, "Data"=[]} ("Data to Send"), "Identifier"=w439, "Data"=w438) -> (w434:T20)
                n133 = Enqueue Element(queue=w433, element=w434, error in (no error)=w437) -> (error out=w436:errorcluster)  [unwired: 3 out]
              }
            }
          }
        }
      }
    }
    frame "TP.CM - CTS" {
      n134 = call-poly "Connection Mode Generation.vi"("ref in"=w444, "State"=TP_Connections_List_State."Get", "error in (no error)"=w454) -> ("ref out"=w443:T5, "Connections"=w445:T28[], "error out"=w446:errorcluster)  [unwired: 2 in, 8 out]
      n135 = call-poly "Connection Mode Generation.vi"("Connections"=w445, "CAN frame"=w442, "error in (no error)"=w446) -> ("Connection Cluster"=w449:T28, "CAN frame out"=w452:T9, "Found?"=w451:bool, "Index"=w450:i32, "error out"=w448:errorcluster)  [unwired: 1 in, 7 out]
      n136 = case shown="False" w451 {
        tunnel: w448 -> [w463 w484]
        tunnel: w449 -> [_ w483]
        tunnel: [w458 w480] -> w453
        tunnel: w450 -> [_ w478]
        tunnel: w452 -> [w461 w477]
        tunnel: w443 -> [_ w476]
        tunnel: w441 -> [w462 _]
        frame False {
          n137 = call-poly "Connnection Mode Buffer.vi"("ref in"=w462, "State"=TP_Connections_List_State."Get", "error in (no error)"=w463) -> ("ref out"=w455:T4, "Connections"=w465:T27[], "error out"=w466:errorcluster)  [unwired: 2 in, 8 out]
          n138 = call-poly "Connnection Mode Buffer.vi"("Connecctions"=w465, "CAN frame"=w461, "error in (no error)"=w466) -> ("Connection Cluster Out"=w456:T27, "Found?"=w460:bool, "Index"=w457:i32, "error out"=w459:errorcluster)  [unwired: 9 out]
          n139 = case shown="False" w460 {
            tunnel: w459 -> [w467 w475]
            tunnel: [w467 w474] -> w458
            tunnel: w457 -> [_ w473]
            tunnel: w456 -> [_ w470]
            tunnel: w455 -> [_ w472]
            frame False {
            }
            frame True {
              n140 = call "Tick Count"() -> ("Tick Count(mSec)"=w468:u32)
              n141 = Bundle By Name(cluster=w470, "Start Time"=w468) -> (w469:T27)
              n142 = call-poly "Connnection Mode Buffer.vi"("Connection Cluster"=w469, "ref in"=w472, "State"=TP_Connections_List_State."Update", "index"=w473, "error in (no error)"=w475) -> ("error out"=w474:errorcluster)  [unwired: 10 out]
            }
          }
        }
        frame True {
          n143 = call-poly "Connection Mode Generation.vi"("Connection Cluster"=w483, "CAN frame"=w477, "error in (no error)"=w484) -> ("Connection Cluster Out"=w482:T28, "error out"=w481:errorcluster)  [unwired: 11 out]
          n144 = call-poly "Connection Mode Generation.vi"("Connection Cluster"=w482, "ref in"=w476, "State"=TP_Connections_List_State."Update", "index"=w478, "error in (no error)"=w481) -> ("error out"=w480:errorcluster)  [unwired: 10 out]
        }
      }
    }
    frame "TP.CM - EndofMsgACK" {
      # "DLE NOTE - Technically, I should wait for this when acquiring a connection mode message from an address other than mine (I generate the message if my address is the one the message is intended for)."
      n145 = call-poly "Connection Mode Generation.vi"("ref in"=w487, "State"=TP_Connections_List_State."Get", "error in (no error)"=w495) -> ("ref out"=w486:T5, "Connections"=w490:T28[], "error out"=w489:errorcluster)  [unwired: 2 in, 8 out]
      n146 = call-poly "Connection Mode Generation.vi"("Connections"=w490, "CAN frame"=w485, "error in (no error)"=w489) -> ("Found?"=w492:bool, "Index"=w493:i32, "error out"=w491:errorcluster)  [unwired: 1 in, 9 out]
      n147 = case shown="True" w492 {
        tunnel: w491 -> [w496 w501]
        tunnel: [w496 w500] -> w494
        tunnel: w493 -> [_ w498]
        tunnel: w486 -> [_ w497]
        frame False {
        }
        frame True {
          n148 = call-poly "Connection Mode Generation.vi"("ref in"=w497, "State"=TP_Connections_List_State."Remove", "index"=w498, "error in (no error)"=w501) -> ("error out"=w500:errorcluster)  [unwired: 1 in, 10 out]
        }
      }
    }
    frame "TP.CM - Abort" {
      n149 = call-poly "Connnection Mode Buffer.vi"("ref in"=w505, "State"=TP_Connections_List_State."Get", "error in (no error)"=w511) -> ("ref out"=w504:T4, "Connections"=w508:T27[], "error out"=w510:errorcluster)  [unwired: 2 in, 8 out]
      n150 = call-poly "Connnection Mode Buffer.vi"("Connecctions"=w508, "CAN frame"=w502, "error in (no error)"=w510) -> ("Found?"=w507:bool, "Index"=w506:i32, "error out"=w513:errorcluster)  [unwired: 1 in, 9 out]
      n151 = case shown="True" w507 {
        tunnel: w513 -> [w523 w535]
        tunnel: [w524 w534] -> w512
        tunnel: w506 -> [_ w532]
        tunnel: w502 -> [w522 _]
        tunnel: w504 -> [_ w531]
        tunnel: w503 -> [w515 _]
        frame False {
          n152 = call-poly "Connection Mode Generation.vi"("ref in"=w515, "State"=TP_Connections_List_State."Get", "error in (no error)"=w523) -> ("ref out"=w514:T5, "Connections"=w518:T28[], "error out"=w517:errorcluster)  [unwired: 2 in, 8 out]
          n153 = call-poly "Connection Mode Generation.vi"("Connections"=w518, "CAN frame"=w522, "error in (no error)"=w517) -> ("Found?"=w520:bool, "Index"=w521:i32, "error out"=w519:errorcluster)  [unwired: 1 in, 9 out]
          n154 = case shown="True" w520 {
            tunnel: w519 -> [w525 w530]
            tunnel: [w525 w529] -> w524
            tunnel: w521 -> [_ w527]
            tunnel: w514 -> [_ w526]
            frame False {
            }
            frame True {
              n155 = call-poly "Connection Mode Generation.vi"("ref in"=w526, "State"=TP_Connections_List_State."Remove", "index"=w527, "error in (no error)"=w530) -> ("error out"=w529:errorcluster)  [unwired: 1 in, 10 out]
            }
          }
        }
        frame True {
          n156 = call-poly "Connnection Mode Buffer.vi"("ref in"=w531, "State"=TP_Connections_List_State."Remove", "index"=w532, "error in (no error)"=w535) -> ("error out"=w534:errorcluster)  [unwired: 1 in, 10 out]
        }
      }
    }
    frame "ACL" {
      # "DLE NOTE - This needs to be added to handle rejections."
      # "Address Claimed (ACL) Stub"
      n157 = Unbundle By Name(w538) -> ("identifier"=w539:u32, "payload"=w546:u8[])
      n158 = call-poly "Common Conversions.vi"("Arb ID"=w539) -> ("Source Address"=w536:u8)  [unwired: 11 in, 3 out]
      n159 = case shown="0..253" w536 {
        selector: w536 -> [_ w550]
        tunnel: w547 -> [w548 w555]
        tunnel: [w548 w549] -> w541
        tunnel: w546 -> [_ w553]
        tunnel: w545 -> [_ w551]
        frame Default {
        }
        frame 0..253 {
          n160 = Bundle By Name(cluster=T23 {"Name"=[], "Address"=0} ("Data"), "Address"=w550, "Name"=w553) -> (w552:T23)
          n161 = call "Network Address Lookup Table.vi"("Action"=Address_Lookup_Table_Action."Add", "error in (no error)"=w555, "Address"=w550, "Data"=w552, "ref in"=w551) -> ("error out"=w549:errorcluster)  [unwired: 3 in, 3 out]
        }
      }
      n162 = And(x=w539, y=u32 536870911) -> (x .and. y?=w542:u32)
      n163 = Bundle By Name(cluster=w538, "identifier"=w542) -> (w543:T9)
      n164 = Enqueue Element(queue=w537, element=w543, error in (no error)=w541) -> (error out=w540:errorcluster)  [unwired: 3 out]
    }
    frame "PDU 2", "Proprietary B" {
      # "Global PDUs (PDU2)"
      n165 = Unbundle By Name(w557) -> ("identifier"=w564:u32)
      n166 = And(x=w564, y=u32 536870911) -> (x .and. y?=w561:u32)
      n167 = Bundle By Name(cluster=w557, "identifier"=w561) -> (w562:T9)
      n168 = Enqueue Element(queue=w558, element=w562, error in (no error)=w559) -> (error out=w560:errorcluster)  [unwired: 3 out]
    }
    frame "TP.CM - Error", "Error" {
      # "Proprietary B Stub"
    }
  }
  "error out" <- w19
